vi "sub_FEA_Make_M_and K_Matrices_LEMP2.vi"(1 "Mode Count":i32, 2 "Setup Parameters":T2) -> (0 "Beam Model":T1)   [LabVIEW 2019]
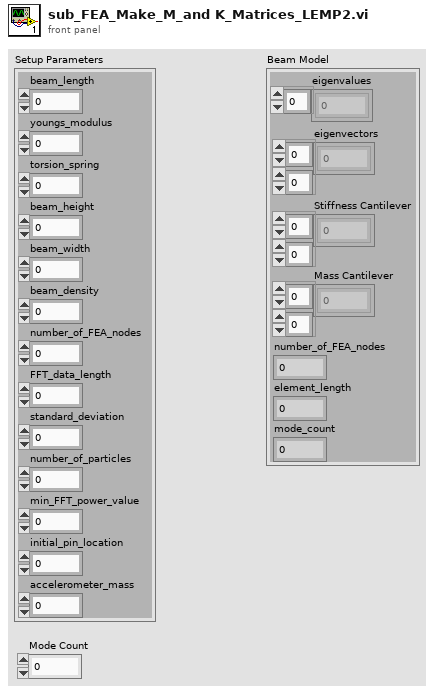
[diagram p1: front panel]
types:
  T1 = cluster{"eigenvalues":dbl[], "element_length ":dbl, "number_of_FEA_nodes":i32, "Stiffness Cantilever":dbl[][], "Mass Cantilever":dbl[][], "eigenvectors":dbl[][], "mode_count":i32}
  T2 = cluster{"beam_length":dbl, "youngs_modulus":dbl, "torsion_spring":dbl, "beam_height":dbl, "beam_width":dbl, "beam_density":dbl, "number_of_FEA_nodes":i32, "FFT_data_length":i32, "standard_deviation":dbl, "number_of_particles":i32, "min_FFT_power_value":dbl, "initial_pin_location":i32, "accelerometer_mass":dbl}
  T3 = cluster{"eigenvalues":dbl[], "element_length ":dbl, "number_of_FEA_nodes":i32, "Stiffness Cantilever":dbl[][], "Mass Cantilever":dbl[][], "eigenvectors":dbl[][], "Mode Count":i32}
  T4 = typedef "NI_Matrix.lvlib/RealMatrix.ctl" = dbl[][]
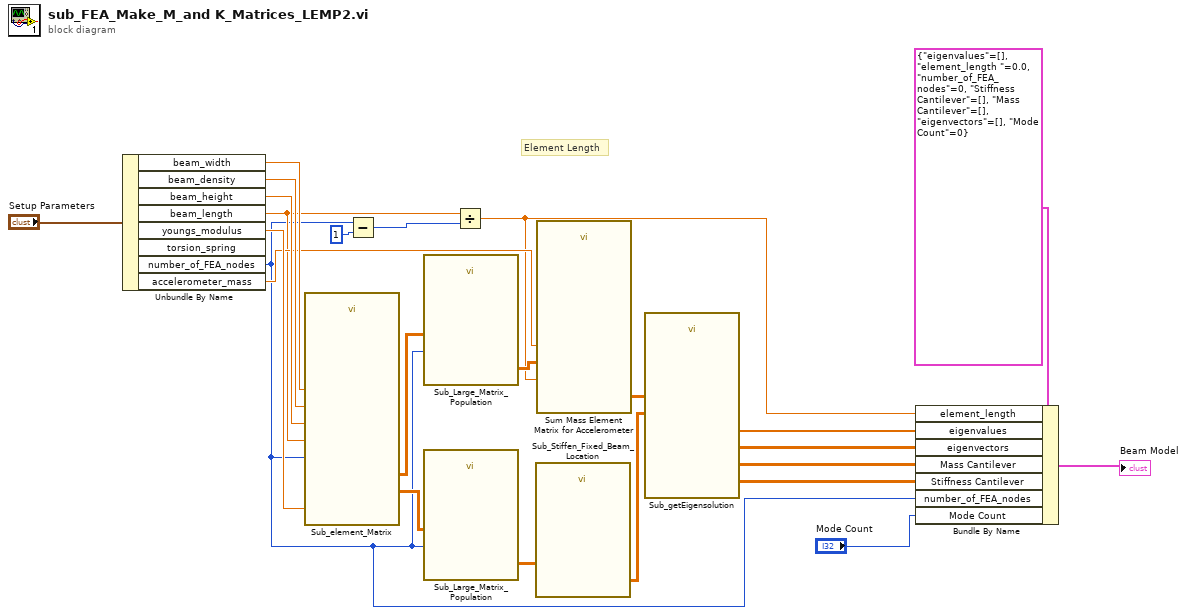
[diagram p0: block diagram]
diagram:
  # "Element Length"
  n1 = Unbundle By Name("Setup Parameters") -> ("beam_width"=w19:dbl, "beam_density"=w20:dbl, "beam_height"=w21:dbl, "beam_length"=w13:dbl, "youngs_modulus"=w22:dbl, "number_of_FEA_nodes"=w3:i32, "accelerometer_mass"=w14:dbl)  [unwired: 1 out]
  n2 = call "Sub_element_Matrix.vi"("Length of Beam"=w13, "Young's Modulus"=w22, "No. of Nodes"=w3, "Height"=w21, "Width"=w19, "Density"=w20) -> ("M Element Matrix"=w23:dbl[][], "K Element Matrix"=w24:dbl[][])  [unwired: 11 in, 1 out]
  n3 = Subtract(x=w3, y=1) -> (x-y=w17:i32)
  n4 = call "Sub_Large_Matrix_Population.vi"("No. of Nodes"=w3, "Element Matrix"=w23) -> ("Matrix w/o BC"=w18:dbl[][])  [unwired: 9 in]
  n5 = call "Sub_Large_Matrix_Population.vi"("No. of Nodes"=w3, "Element Matrix"=w24) -> ("Matrix w/o BC"=w12:dbl[][])  [unwired: 9 in]
  n6 = Divide(x=w13, y=w17) -> (x/y=w8:dbl)
  n7 = call "Sub_Stiffen_Fixed_Beam_Location.vi"("Pre-BC Matrix"=w12) -> ("Post-BC Matrix"=w10:dbl[][])  [unwired: 10 in]
  n8 = call "Sum Mass Element Matrix for Accelerometer.vi"("Matrix w/o BC"=w18, "accelerometer_mass"=w14, "Element Length"=w8) -> ("Matrix W/ Accelerometer"=w11:dbl[][])  [unwired: 8 in]
  n9 = call "Sub_getEigensolution.vi"("MASS"=w11, "STIFF"=w10) -> ("MASS"=w5:T4, "STIFF"=w4:T4, "Eigenvectors"=w6:T4, "Eigenvalues"=w7:cdb[])  [unwired: 6 in]
  n10 = Bundle By Name(cluster=T3 {"eigenvalues"=[], "element_length "=0.0, "number_of_FEA_nodes"=0, "Stiffness Cantilever"=[], "Mass Cantilever"=[], "eigenvectors"=[], "Mode Count"=0} ("Setup Parameters"), "element_length"=w8, "eigenvalues"=w7, "eigenvectors"=w6, "Mass Cantilever"=w5, "Stiffness Cantilever"=w4, "number_of_FEA_nodes"=w3, "Mode Count"="Mode Count") -> (→"Beam Model":T3)
